vi "Final Harmonics.vi"(0 "Header File Input":string[][](array[string])=[["Instrument", "YOKOGAWA,WT332,C2QB17128V,F1.03\n"], ["Instr Driver Revision", "1.0 F1.03"], ["Start Time", "1.0"], ["Voltage Range", "6/1/2015 11:50 AM"], ["Current Range", "Auto"], ["Update Rate", "Auto"], ["Standard", "0.250"], ["Algorithm", "IEC62301 Ed.2(Auto)"], ["Stop Factor", "Linear Regression"], ["Valid Period", ""], ["Start Total Harmonic Distortion Uthd 1", "0.065"], ["Start Total Harmonic Distortion Uthd 2", ""], ["End Total Harmonic Distortion Uthd 1", ""], ["End Total Harmonic Distortion Uthd 2", ""], ["Max Power (Watts)", ""], ["Power Variation (%)", ""], ["", ""]], 1 "Error Output?":bool=TRUE, 5 "Standby Power In 2":T2={"Standby Power Spreadsheet"=[], "Standby Power - Pia (Watts)"=0.0, "Off Mode Power - Poff (Watts)"=0.0, "Sia hr/yr"=8620.0, "Soff hr/yr"=0.0, "Yearly Energy Etso kWh/yr"=0.0, "Maximum Power (Watts)"=0.0, "Power Variation (%)"=0.0, "Slope (mW/hr)"=0.0, "Final Harmonics-U1 (%)"="", "Final Harmonics-U2 (%)"="", "Energy (Wh)"=0.0}, 7 "Elapsed Time.":dbl, 9 "Appliance Common":T1, 11 "error in (no error)":errorcluster) -> (4 "Header File Output":string[][](array[string]), 6 "Standby Power Out":T2={"Standby Power Spreadsheet"=[], "Standby Power - Pia (Watts)"=0.0, "Off Mode Power - Poff (Watts)"=0.0, "Sia hr/yr"=8620.0, "Soff hr/yr"=0.0, "Yearly Energy Etso kWh/yr"=0.0, "Maximum Power (Watts)"=0.0, "Power Variation (%)"=0.0, "Slope (mW/hr)"=0.0, "Final Harmonics-U1 (%)"="", "Final Harmonics-U2 (%)"="", "Energy (Wh)"=0.0}, 15 "error out":errorcluster)   [LabVIEW 2018]
uses:
  Type Definitions/Standby Power Main Data.ctl
  Washer DOE/Type Definitions/DOE Appliance Common.ctl
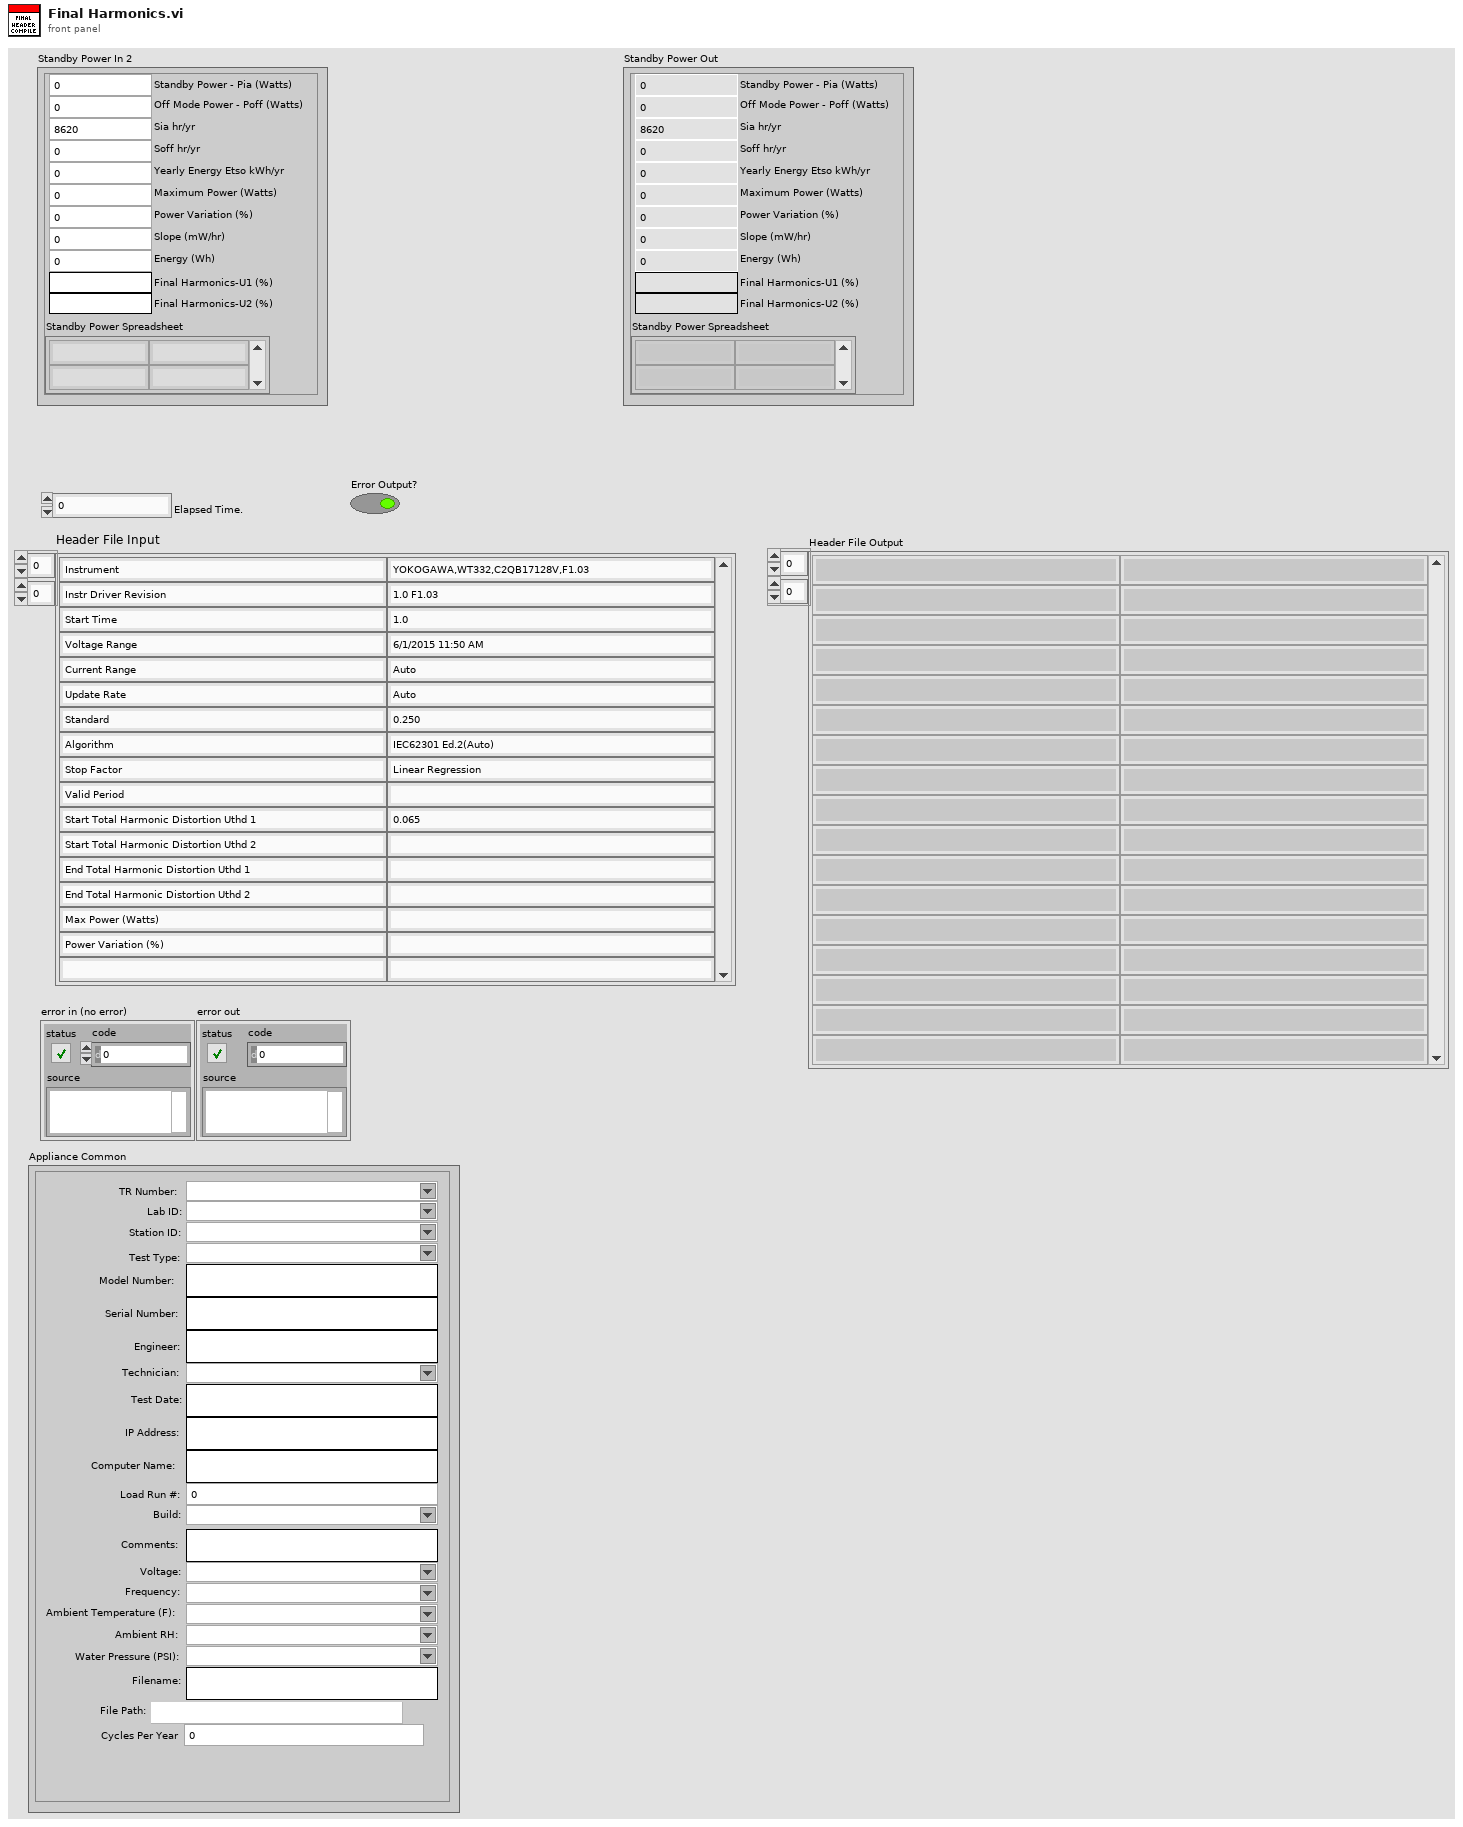
[diagram p1: front panel]
types:
  T1 = typedef "DOE Appliance Common.ctl" = cluster{"Engineer:":string, "Model Number:":string, "Serial Number:":string, "Comments:":string, "Station ID:":string, "Technician:":string, "TR Number:":string, "Lab ID:":string, "Voltage:":string, "Water Pressure (PSI):":string, "Test Date:":string, "Computer Name:":string, "IP Address:":string, "Ambient RH:":string, "Frequency:":string, "Build:":string, "Filename:":string, "Test Type:":string, "Load Run #:":i32, "Ambient Temperature (F):":string, "File Path:":path, "Cycles Per Year":u32}
  T2 = typedef "Standby Power Main Data.ctl" = cluster{"Standby Power Spreadsheet":string[][], "Standby Power - Pia (Watts)":dbl, "Off Mode Power - Poff (Watts)":dbl, "Sia hr/yr":dbl, "Soff hr/yr":dbl, "Yearly Energy Etso kWh/yr":dbl, "Maximum Power (Watts)":dbl, "Power Variation (%)":dbl, "Slope (mW/hr)":dbl, "Final Harmonics-U1 (%)":string, "Final Harmonics-U2 (%)":string, "Energy (Wh)":dbl}
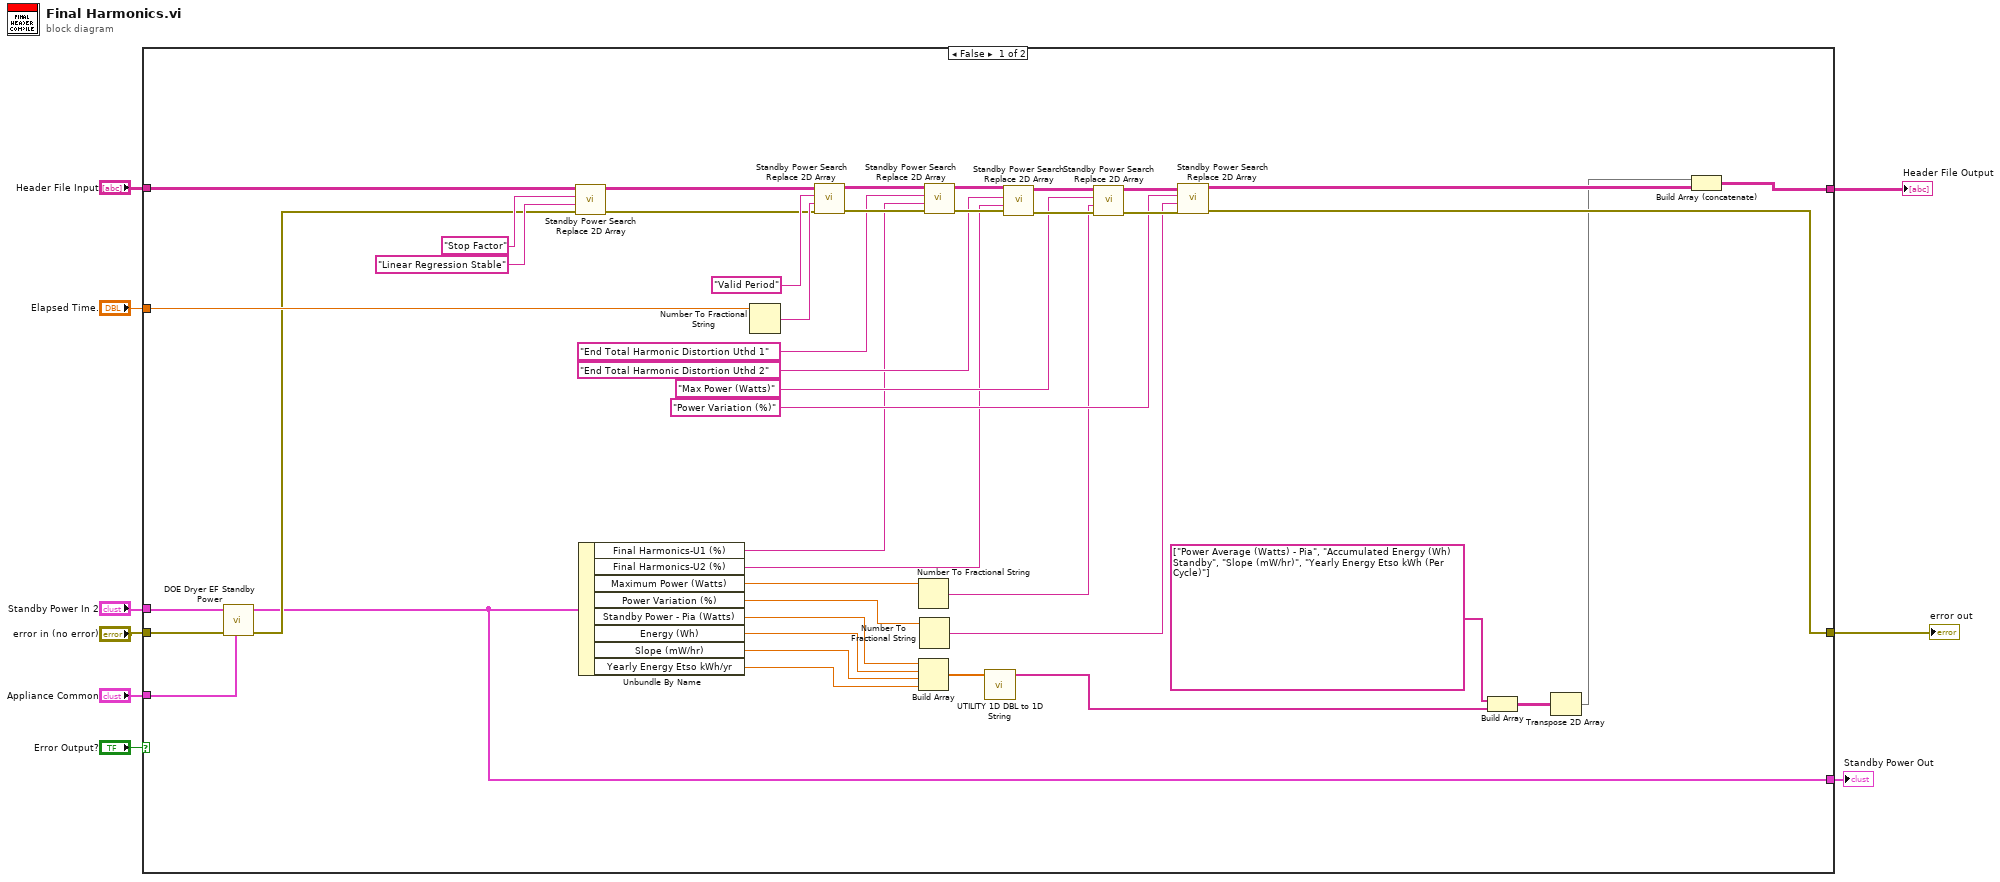
[diagram p0: block diagram]
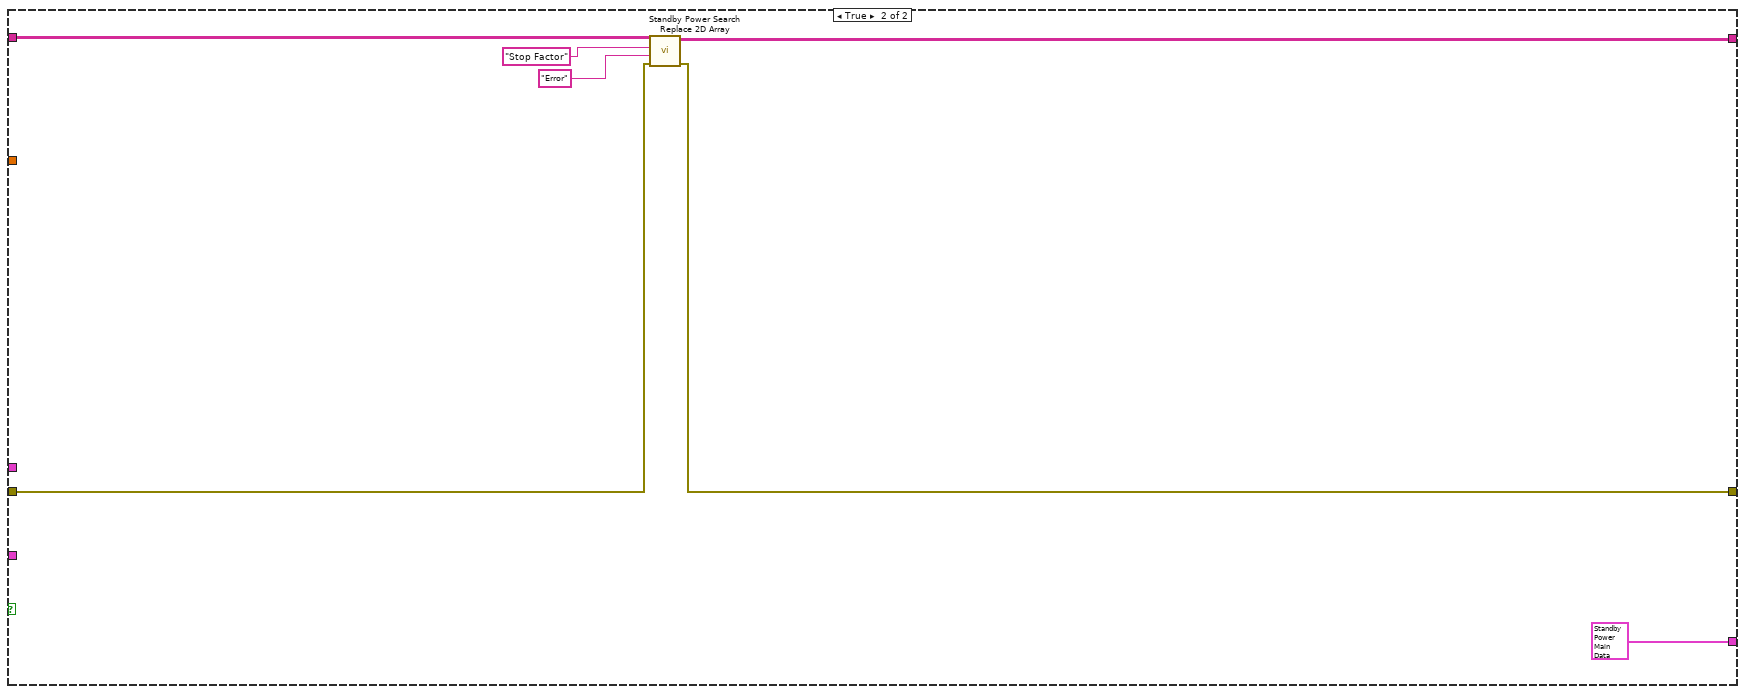
[diagram p2: hidden frame]
diagram:
  n1 = case shown="False" "Error Output?" {
    tunnel: [w24 w57] -> w7
    tunnel: "Header File Input" -> [w51 w59]
    tunnel: [w13 w56] -> w8
    tunnel: "Elapsed Time." -> [w52 _]
    tunnel: "Standby Power In 2" -> [w26 _]
    tunnel: "error in (no error)" -> [w12 w55]
    tunnel: [w11 T2 {"Standby Power Spreadsheet"=[], "Standby Power - Pia (Watts)"=0.0, "Off Mode Power - Poff (Watts)"=0.0, "Sia hr/yr"=8620.0, "Soff hr/yr"=0.0, "Yearly Energy Etso kWh/yr"=0.0, "Maximum Power (Watts)"=0.0, "Power Variation (%)"=0.0, "Slope (mW/hr)"=0.0, "Final Harmonics-U1 (%)"="", "Final Harmonics-U2 (%)"="", "Energy (Wh)"=0.0} ("Standby Power Out")] -> w2
    tunnel: "Appliance Common" -> [w10 _]
    frame False {
      n2 = call "DOE Dryer EF Standby Power.vi"("Appliance Common"=w10, "Error In"=w12, "Standby Power In"=w26) -> ("Error Out"=w25:errorcluster, "Standby Power Out"=w11:T2)  [unwired: 7 in]
      n3 = call "Standby Power Search Replace 2D Array.vi"("Error In"=w25, "Insert Value"="Linear Regression Stable", "Search Element"="Stop Factor", "Array in in"=w51) -> ("Error Out"=w41:errorcluster, "Array out"=w46:string[][])  [unwired: 6 in]
      n4 = Unbundle By Name(w11) -> ("Final Harmonics-U1 (%)"=w32:string, "Final Harmonics-U2 (%)"=w31:string, "Maximum Power (Watts)"=w30:dbl, "Power Variation (%)"=w28:dbl, "Standby Power - Pia (Watts)"=w23:dbl, "Energy (Wh)"=w20:dbl, "Slope (mW/hr)"=w22:dbl, "Yearly Energy Etso kWh/yr"=w21:dbl)
      n5 = Number To Fractional String(number=w52) -> (F-format string=w47:string)  [unwired: 3 in]
      n6 = call "Standby Power Search Replace 2D Array.vi"("Error In"=w41, "Insert Value"=w47, "Search Element"="Valid Period" ("element"), "Array in in"=w46) -> ("Error Out"=w40:errorcluster, "Array out"=w45:string[][])  [unwired: 6 in]
      n7 = Number To Fractional String(number=w30) -> (F-format string=w29:string)  [unwired: 3 in]
      n8 = Build Array(w23, w20, w22, w21) -> (w19:dbl[])
      n9 = Number To Fractional String(number=w28) -> (F-format string=w27:string)  [unwired: 3 in]
      n10 = call "Standby Power Search Replace 2D Array.vi"("Error In"=w40, "Insert Value"=w32, "Search Element"="End Total Harmonic Distortion Uthd 1" ("element"), "Array in in"=w45) -> ("Error Out"=w39:errorcluster, "Array out"=w44:string[][])  [unwired: 6 in]
      n11 = call "UTILITY 1D DBL to 1D String.vi"("1D DBL"=w19) -> ("1D String"=w17:string[])  [unwired: 10 in]
      n12 = call "Standby Power Search Replace 2D Array.vi"("Error In"=w39, "Insert Value"=w31, "Search Element"="End Total Harmonic Distortion Uthd 2" ("element"), "Array in in"=w44) -> ("Error Out"=w38:errorcluster, "Array out"=w43:string[][])  [unwired: 6 in]
      n13 = call "Standby Power Search Replace 2D Array.vi"("Error In"=w38, "Insert Value"=w29, "Search Element"="Max Power (Watts)" ("element"), "Array in in"=w43) -> ("Error Out"=w37:errorcluster, "Array out"=w42:string[][])  [unwired: 6 in]
      n14 = call "Standby Power Search Replace 2D Array.vi"("Error In"=w37, "Insert Value"=w27, "Search Element"="Power Variation (%)" ("element"), "Array in in"=w42) -> ("Error Out"=w24:errorcluster, "Array out"=w15:string[][])  [unwired: 6 in]
      n15 = Build Array(string[] ["Power Average (Watts) - Pia", "Accumulated Energy (Wh) Standby", "Slope (mW/hr)", "Yearly Energy Etso kWh (Per Cycle)"] ("element"), w17) -> (w16:string[][])
      n16 = Transpose 2D Array(2D array=w16) -> (transposed array=w14:string[][])
      n17 = Build Array (concatenate)(w14, w15) -> (w13:string[][])
    }
    frame True {
      n18 = call "Standby Power Search Replace 2D Array.vi"("Error In"=w55, "Insert Value"="Error" ("Error Note"), "Search Element"="Stop Factor" ("element"), "Array in in"=w59) -> ("Error Out"=w57:errorcluster, "Array out"=w56:string[][])  [unwired: 6 in]
    }
  }
  "Header File Output" <- w8
  "error out" <- w7
  "Standby Power Out" <- w2
